vi "Autonomous Independent.vi"() -> ()   [LabVIEW 2016]
doc: "This VI is called when autonomous begins, and will automatically be terminated when autonomous ends. You can carry out timed or sensor driven robot movement independently without needing to return to the caller."
uses:
  <vilib>/Rock Robotics/Network Tables/NT Read Number.vi
  Global 2.vi
  Systems/Global 1.vi
panel:
  out "Numeric":i32=78
  out "Gyro":dbl=-0.15423582405
  in  "Oscillate effort":dbl=0.25 format="%#_13g"
  out "Auto Mode":dbl=2.0
  in  "Auton_Modes":T1(array[cluster])=[{"Actions"=[{"Effort"=0.55, "Duration"=3.5, "Action"=enum."Vision Correction", "Encoder"=0.0, "Condition"=FALSE}, {"Effort"=0.0, "Duration"=0.0, "Action"=enum."Nothing", "Encoder"=0.0, "Condition"=FALSE}]}, {"Actions"=[{"Effort"=0.53, "Duration"=1.0, "Action"=enum."Shoot", "Encoder"=6.462, "Condition"=TRUE}, {"Effort"=0.0, "Duration"=3.0, "Action"=enum."Index", "Encoder"=0.0, "Condition"=FALSE}, {"Effort"=0.3, "Duration"=2.0, "Action"=enum."Turn", "Encoder"=38.0, "Condition"=FALSE}, {"Effort"=0.3, "Duration"=5.0, "Action"=enum."Drive", "Encoder"=0.0, "Condition"=TRUE}, {"Effort"=0.25, "Duration"=0.0, "Action"=enum."Nothing", "Encoder"=57.0, "Condition"=FALSE}, {"Effort"=-0.25, "Duration"=0.0, "Action"=enum."Nothing", "Encoder"=0.0, "Condition"=FALSE}, {"Effort"=1.0, "Duration"=0.0, "Action"=enum."Nothing", "Encoder"=0.0, "Condition"=FALSE}, {"Effort"=0.25, "Duration"=0.0, "Action"=enum."Nothing", "Encoder"=0.0, "Condition"=FALSE}]}, {"Actions"=[{"Effort"=0.0, "Duration"=0.1, "Action"=enum."Drive Encoder Reset", "Encoder"=0.0, "Condition"=FALSE}, {"Effort"=0.0, "Duration"=0.1, "Action"=enum."Gyro Reset", "Encoder"=0.0, "Condition"=FALSE}, {"Effort"=0.3, "Duration"=2.5, "Action"=enum."Drive", "Encoder"=1000.0, "Condition"=TRUE}, {"Effort"=1.0, "Duration"=1.0, "Action"=enum."Gear0", "Encoder"=0.0, "Condition"=FALSE}, {"Effort"=1.0, "Duration"=0.0, "Action"=enum."Nothing", "Encoder"=0.0, "Condition"=FALSE}, {"Effort"=1.0, "Duration"=0.5, "Action"=enum."Nothing", "Encoder"=0.0, "Condition"=FALSE}, {"Effort"=0.0, "Duration"=0.0, "Action"=enum."Drive Encoder Reset", "Encoder"=0.0, "Condition"=FALSE}, {"Effort"=0.3, "Duration"=0.5, "Action"=enum."Nothing", "Encoder"=24.0, "Condition"=TRUE}, {"Effort"=0.0, "Duration"=0.0, "Action"=enum."Nothing", "Encoder"=0.0, "Condition"=FALSE}, {"Effort"=-0.2, "Duration"=2.0, "Action"=enum."Drive", "Encoder"=1000.0, "Condition"=TRUE}, {"Effort"=0.0, "Duration"=0.0, "Action"=enum."Drive Encoder Reset", "Encoder"=0.0, "Condition"=FALSE}, {"Effort"=-0.25, "Duration"=0.0, "Action"=enum."Nothing", "Encoder"=12.0, "Condition"=FALSE}]}, {"Actions"=[{"Effort"=0.0, "Duration"=0.1, "Action"=enum."Drive Encoder Reset", "Encoder"=6.462, "Condition"=FALSE}, {"Effort"=0.0, "Duration"=0.1, "Action"=enum."Gyro Reset", "Encoder"=0.0, "Condition"=FALSE}, {"Effort"=-0.25, "Duration"=1.0, "Action"=enum."Drive", "Encoder"=6.462, "Condition"=FALSE}, {"Effort"=0.0, "Duration"=0.1, "Action"=enum."Gyro Reset", "Encoder"=0.0, "Condition"=FALSE}, {"Effort"=-0.25, "Duration"=0.0, "Action"=enum."Turn", "Encoder"=0.0, "Condition"=FALSE}, {"Effort"=-0.25, "Duration"=0.0, "Action"=enum."Drive", "Encoder"=7.5, "Condition"=FALSE}, {"Effort"=-1.0, "Duration"=0.0, "Action"=enum."Gear0", "Encoder"=0.0, "Condition"=FALSE}, {"Effort"=0.25, "Duration"=0.0, "Action"=enum."Drive", "Encoder"=3.0, "Condition"=FALSE}]}, {"Actions"=[{"Effort"=0.0, "Duration"=0.1, "Action"=enum."Drive Encoder Reset", "Encoder"=6.462, "Condition"=FALSE}, {"Effort"=0.0, "Duration"=0.1, "Action"=enum."Gyro Reset", "Encoder"=0.0, "Condition"=FALSE}, {"Effort"=-0.25, "Duration"=1.0, "Action"=enum."Drive", "Encoder"=6.462, "Condition"=FALSE}, {"Effort"=0.0, "Duration"=0.1, "Action"=enum."Gyro Reset", "Encoder"=0.0, "Condition"=FALSE}, {"Effort"=-0.25, "Duration"=0.0, "Action"=enum."Turn", "Encoder"=0.0, "Condition"=FALSE}, {"Effort"=-0.25, "Duration"=0.0, "Action"=enum."Drive", "Encoder"=7.5, "Condition"=FALSE}, {"Effort"=-1.0, "Duration"=0.0, "Action"=enum."Gear0", "Encoder"=0.0, "Condition"=FALSE}, {"Effort"=0.25, "Duration"=0.0, "Action"=enum."Drive", "Encoder"=3.0, "Condition"=FALSE}]}, {"Actions"=[{"Effort"=0.0, "Duration"=0.1, "Action"=enum."Drive Encoder Reset", "Encoder"=0.0, "Condition"=FALSE}, {"Effort"=0.0, "Duration"=0.1, "Action"=enum."Gyro Reset", "Encoder"=0.0, "Condition"=FALSE}, {"Effort"=0.25, "Duration"=1.0, "Action"=enum."Drive", "Encoder"=6.462, "Condition"=FALSE}, {"Effort"=1.0, "Duration"=0.1, "Action"=enum."Gyro Reset", "Encoder"=0.0, "Condition"=FALSE}, {"Effort"=0.25, "Duration"=0.0, "Action"=enum."Turn", "Encoder"=0.0, "Condition"=FALSE}, {"Effort"=0.25, "Duration"=0.0, "Action"=enum."Drive", "Encoder"=7.5, "Condition"=FALSE}, {"Effort"=1.0, "Duration"=0.0, "Action"=enum."Gear0", "Encoder"=0.0, "Condition"=FALSE}, {"Effort"=-0.25, "Duration"=0.0, "Action"=enum."Drive", "Encoder"=3.0, "Condition"=FALSE}]}, {"Actions"=[{"Effort"=0.0, "Duration"=0.1, "Action"=enum."Nothing", "Encoder"=0.0, "Condition"=FALSE}, {"Effort"=0.0, "Duration"=0.1, "Action"=enum."Gyro Reset", "Encoder"=0.0, "Condition"=FALSE}, {"Effort"=0.25, "Duration"=5.0, "Action"=enum."Drive", "Encoder"=60000.0, "Condition"=TRUE}, {"Effort"=0.75, "Duration"=1.0, "Action"=enum."Nothing", "Encoder"=0.0, "Condition"=FALSE}, {"Effort"=0.0, "Duration"=1.0, "Action"=enum."Nothing", "Encoder"=0.0, "Condition"=FALSE}, {"Effort"=0.0, "Duration"=0.0, "Action"=enum."Nothing", "Encoder"=0.0, "Condition"=FALSE}]}, {"Actions"=[{"Effort"=0.0, "Duration"=0.5, "Action"=enum."Drive Encoder Reset", "Encoder"=0.0, "Condition"=FALSE}, {"Effort"=0.55, "Duration"=4.25, "Action"=enum."Gyro Reset", "Encoder"=0.0, "Condition"=FALSE}, {"Effort"=-0.5, "Duration"=0.0, "Action"=enum."Drive", "Encoder"=46.0, "Condition"=FALSE}, {"Effort"=0.3, "Duration"=1.0, "Action"=enum."Nothing", "Encoder"=0.0, "Condition"=FALSE}, {"Effort"=0.3, "Duration"=2.0, "Action"=enum."Vision Correction", "Encoder"=76.6, "Condition"=FALSE}, {"Effort"=-0.25, "Duration"=1.0, "Action"=enum."Drive", "Encoder"=18.5, "Condition"=TRUE}, {"Effort"=1.0, "Duration"=0.0, "Action"=enum."Gear0", "Encoder"=0.0, "Condition"=FALSE}, {"Effort"=0.3, "Duration"=1.3, "Action"=enum."Drive", "Encoder"=30.0, "Condition"=TRUE}, {"Effort"=0.0, "Duration"=0.0, "Action"=enum."Nothing", "Encoder"=0.0, "Condition"=FALSE}, {"Effort"=0.03, "Duration"=0.0, "Action"=enum."Turn", "Encoder"=0.0, "Condition"=FALSE}, {"Effort"=0.0, "Duration"=0.0, "Action"=enum."Drive", "Encoder"=0.0, "Condition"=FALSE}]}, {"Actions"=[{"Effort"=0.0, "Duration"=0.0, "Action"=enum."Nothing", "Encoder"=0.0, "Condition"=FALSE}]}, {"Actions"=[{"Effort"=0.0, "Duration"=2.5, "Action"=enum."Shoot", "Encoder"=0.0, "Condition"=FALSE}, {"Effort"=0.0, "Duration"=5.0, "Action"=enum."Index", "Encoder"=0.0, "Condition"=FALSE}, {"Effort"=0.25, "Duration"=3.5, "Action"=enum."Nothing", "Encoder"=88.0, "Condition"=FALSE}, {"Effort"=1.0, "Duration"=1.0, "Action"=enum."Nothing", "Encoder"=0.0, "Condition"=FALSE}, {"Effort"=1.0, "Duration"=1.0, "Action"=enum."Nothing", "Encoder"=0.0, "Condition"=FALSE}, {"Effort"=1.0, "Duration"=0.5, "Action"=enum."Nothing", "Encoder"=0.0, "Condition"=FALSE}, {"Effort"=0.0, "Duration"=0.0, "Action"=enum."Nothing", "Encoder"=0.0, "Condition"=FALSE}, {"Effort"=-0.25, "Duration"=0.0, "Action"=enum."Nothing", "Encoder"=3.0, "Condition"=FALSE}, {"Effort"=0.0, "Duration"=0.0, "Action"=enum."Nothing", "Encoder"=0.0, "Condition"=FALSE}, {"Effort"=0.25, "Duration"=0.0, "Action"=enum."Nothing", "Encoder"=24.0, "Condition"=FALSE}, {"Effort"=0.0, "Duration"=0.0, "Action"=enum."Nothing", "Encoder"=0.0, "Condition"=FALSE}, {"Effort"=-0.25, "Duration"=0.0, "Action"=enum."Nothing", "Encoder"=12.0, "Condition"=FALSE}]}, {"Actions"=[{"Effort"=0.0, "Duration"=0.1, "Action"=enum."Drive Encoder Reset", "Encoder"=0.0, "Condition"=FALSE}, {"Effort"=0.0, "Duration"=1.0, "Action"=enum."Gyro Reset", "Encoder"=0.0, "Condition"=FALSE}, {"Effort"=0.3, "Duration"=1.4, "Action"=enum."Drive", "Encoder"=88.0, "Condition"=TRUE}, {"Effort"=0.3, "Duration"=4.0, "Action"=enum."Turn", "Encoder"=2.0, "Condition"=FALSE}, {"Effort"=1.0, "Duration"=1.0, "Action"=enum."Nothing", "Encoder"=0.0, "Condition"=FALSE}, {"Effort"=1.0, "Duration"=0.5, "Action"=enum."Nothing", "Encoder"=0.0, "Condition"=FALSE}, {"Effort"=0.0, "Duration"=0.0, "Action"=enum."Nothing", "Encoder"=0.0, "Condition"=FALSE}, {"Effort"=-0.25, "Duration"=0.0, "Action"=enum."Nothing", "Encoder"=3.0, "Condition"=FALSE}, {"Effort"=0.0, "Duration"=0.0, "Action"=enum."Nothing", "Encoder"=0.0, "Condition"=FALSE}, {"Effort"=0.25, "Duration"=0.0, "Action"=enum."Nothing", "Encoder"=24.0, "Condition"=FALSE}, {"Effort"=0.0, "Duration"=0.0, "Action"=enum."Nothing", "Encoder"=0.0, "Condition"=FALSE}, {"Effort"=-0.25, "Duration"=0.0, "Action"=enum."Nothing", "Encoder"=12.0, "Condition"=FALSE}]}, {"Actions"=[{"Effort"=0.0, "Duration"=1.0, "Action"=enum."Drive Encoder Reset", "Encoder"=0.0, "Condition"=FALSE}, {"Effort"=0.0, "Duration"=1.0, "Action"=enum."Shoot", "Encoder"=0.0, "Condition"=FALSE}, {"Effort"=0.25, "Duration"=5.0, "Action"=enum."Index", "Encoder"=88.0, "Condition"=FALSE}, {"Effort"=1.0, "Duration"=1.0, "Action"=enum."Nothing", "Encoder"=0.0, "Condition"=FALSE}, {"Effort"=1.0, "Duration"=1.0, "Action"=enum."Nothing", "Encoder"=0.0, "Condition"=FALSE}, {"Effort"=1.0, "Duration"=0.5, "Action"=enum."Nothing", "Encoder"=0.0, "Condition"=FALSE}, {"Effort"=0.0, "Duration"=0.0, "Action"=enum."Nothing", "Encoder"=0.0, "Condition"=FALSE}, {"Effort"=-0.25, "Duration"=0.0, "Action"=enum."Nothing", "Encoder"=3.0, "Condition"=FALSE}, {"Effort"=0.0, "Duration"=0.0, "Action"=enum."Nothing", "Encoder"=0.0, "Condition"=FALSE}, {"Effort"=0.25, "Duration"=0.0, "Action"=enum."Nothing", "Encoder"=24.0, "Condition"=FALSE}, {"Effort"=0.0, "Duration"=0.0, "Action"=enum."Nothing", "Encoder"=0.0, "Condition"=FALSE}, {"Effort"=-0.25, "Duration"=0.0, "Action"=enum."Nothing", "Encoder"=12.0, "Condition"=FALSE}]}, {"Actions"=[{"Effort"=0.0, "Duration"=0.1, "Action"=enum."Drive Encoder Reset", "Encoder"=0.0, "Condition"=FALSE}, {"Effort"=0.0, "Duration"=1.0, "Action"=enum."Gyro Reset", "Encoder"=0.0, "Condition"=FALSE}, {"Effort"=0.3, "Duration"=1.4, "Action"=enum."Drive", "Encoder"=88.0, "Condition"=TRUE}, {"Effort"=0.3, "Duration"=4.0, "Action"=enum."Turn", "Encoder"=0.0, "Condition"=FALSE}, {"Effort"=1.0, "Duration"=1.0, "Action"=enum."Nothing", "Encoder"=0.0, "Condition"=FALSE}, {"Effort"=1.0, "Duration"=0.5, "Action"=enum."Nothing", "Encoder"=0.0, "Condition"=FALSE}, {"Effort"=0.0, "Duration"=0.0, "Action"=enum."Nothing", "Encoder"=0.0, "Condition"=FALSE}, {"Effort"=0.3, "Duration"=0.5, "Action"=enum."Nothing", "Encoder"=24.0, "Condition"=TRUE}, {"Effort"=0.0, "Duration"=0.0, "Action"=enum."Nothing", "Encoder"=0.0, "Condition"=FALSE}, {"Effort"=-0.2, "Duration"=2.0, "Action"=enum."Nothing", "Encoder"=24.0, "Condition"=TRUE}, {"Effort"=0.0, "Duration"=0.0, "Action"=enum."Nothing", "Encoder"=0.0, "Condition"=FALSE}, {"Effort"=-0.25, "Duration"=0.0, "Action"=enum."Nothing", "Encoder"=12.0, "Condition"=FALSE}]}]
  # "Nothing"
  # "Boiler Right Right side gear"
  # "Middle Gear"
  # "Boiler Right Left Side Gear"
  # "Boiler Left RightSide Gear"
  # "Boiler Left Left Side Gear"
  # "Drive"
  # "Vision Correction"
  # "Hopper"
  # "10 ball"
  # "Farside"
  # "Boilerside-10 ball"
  # "Auto 5"
  # "Auto 6"
  # "Auto 6"
  # "Auto 7"
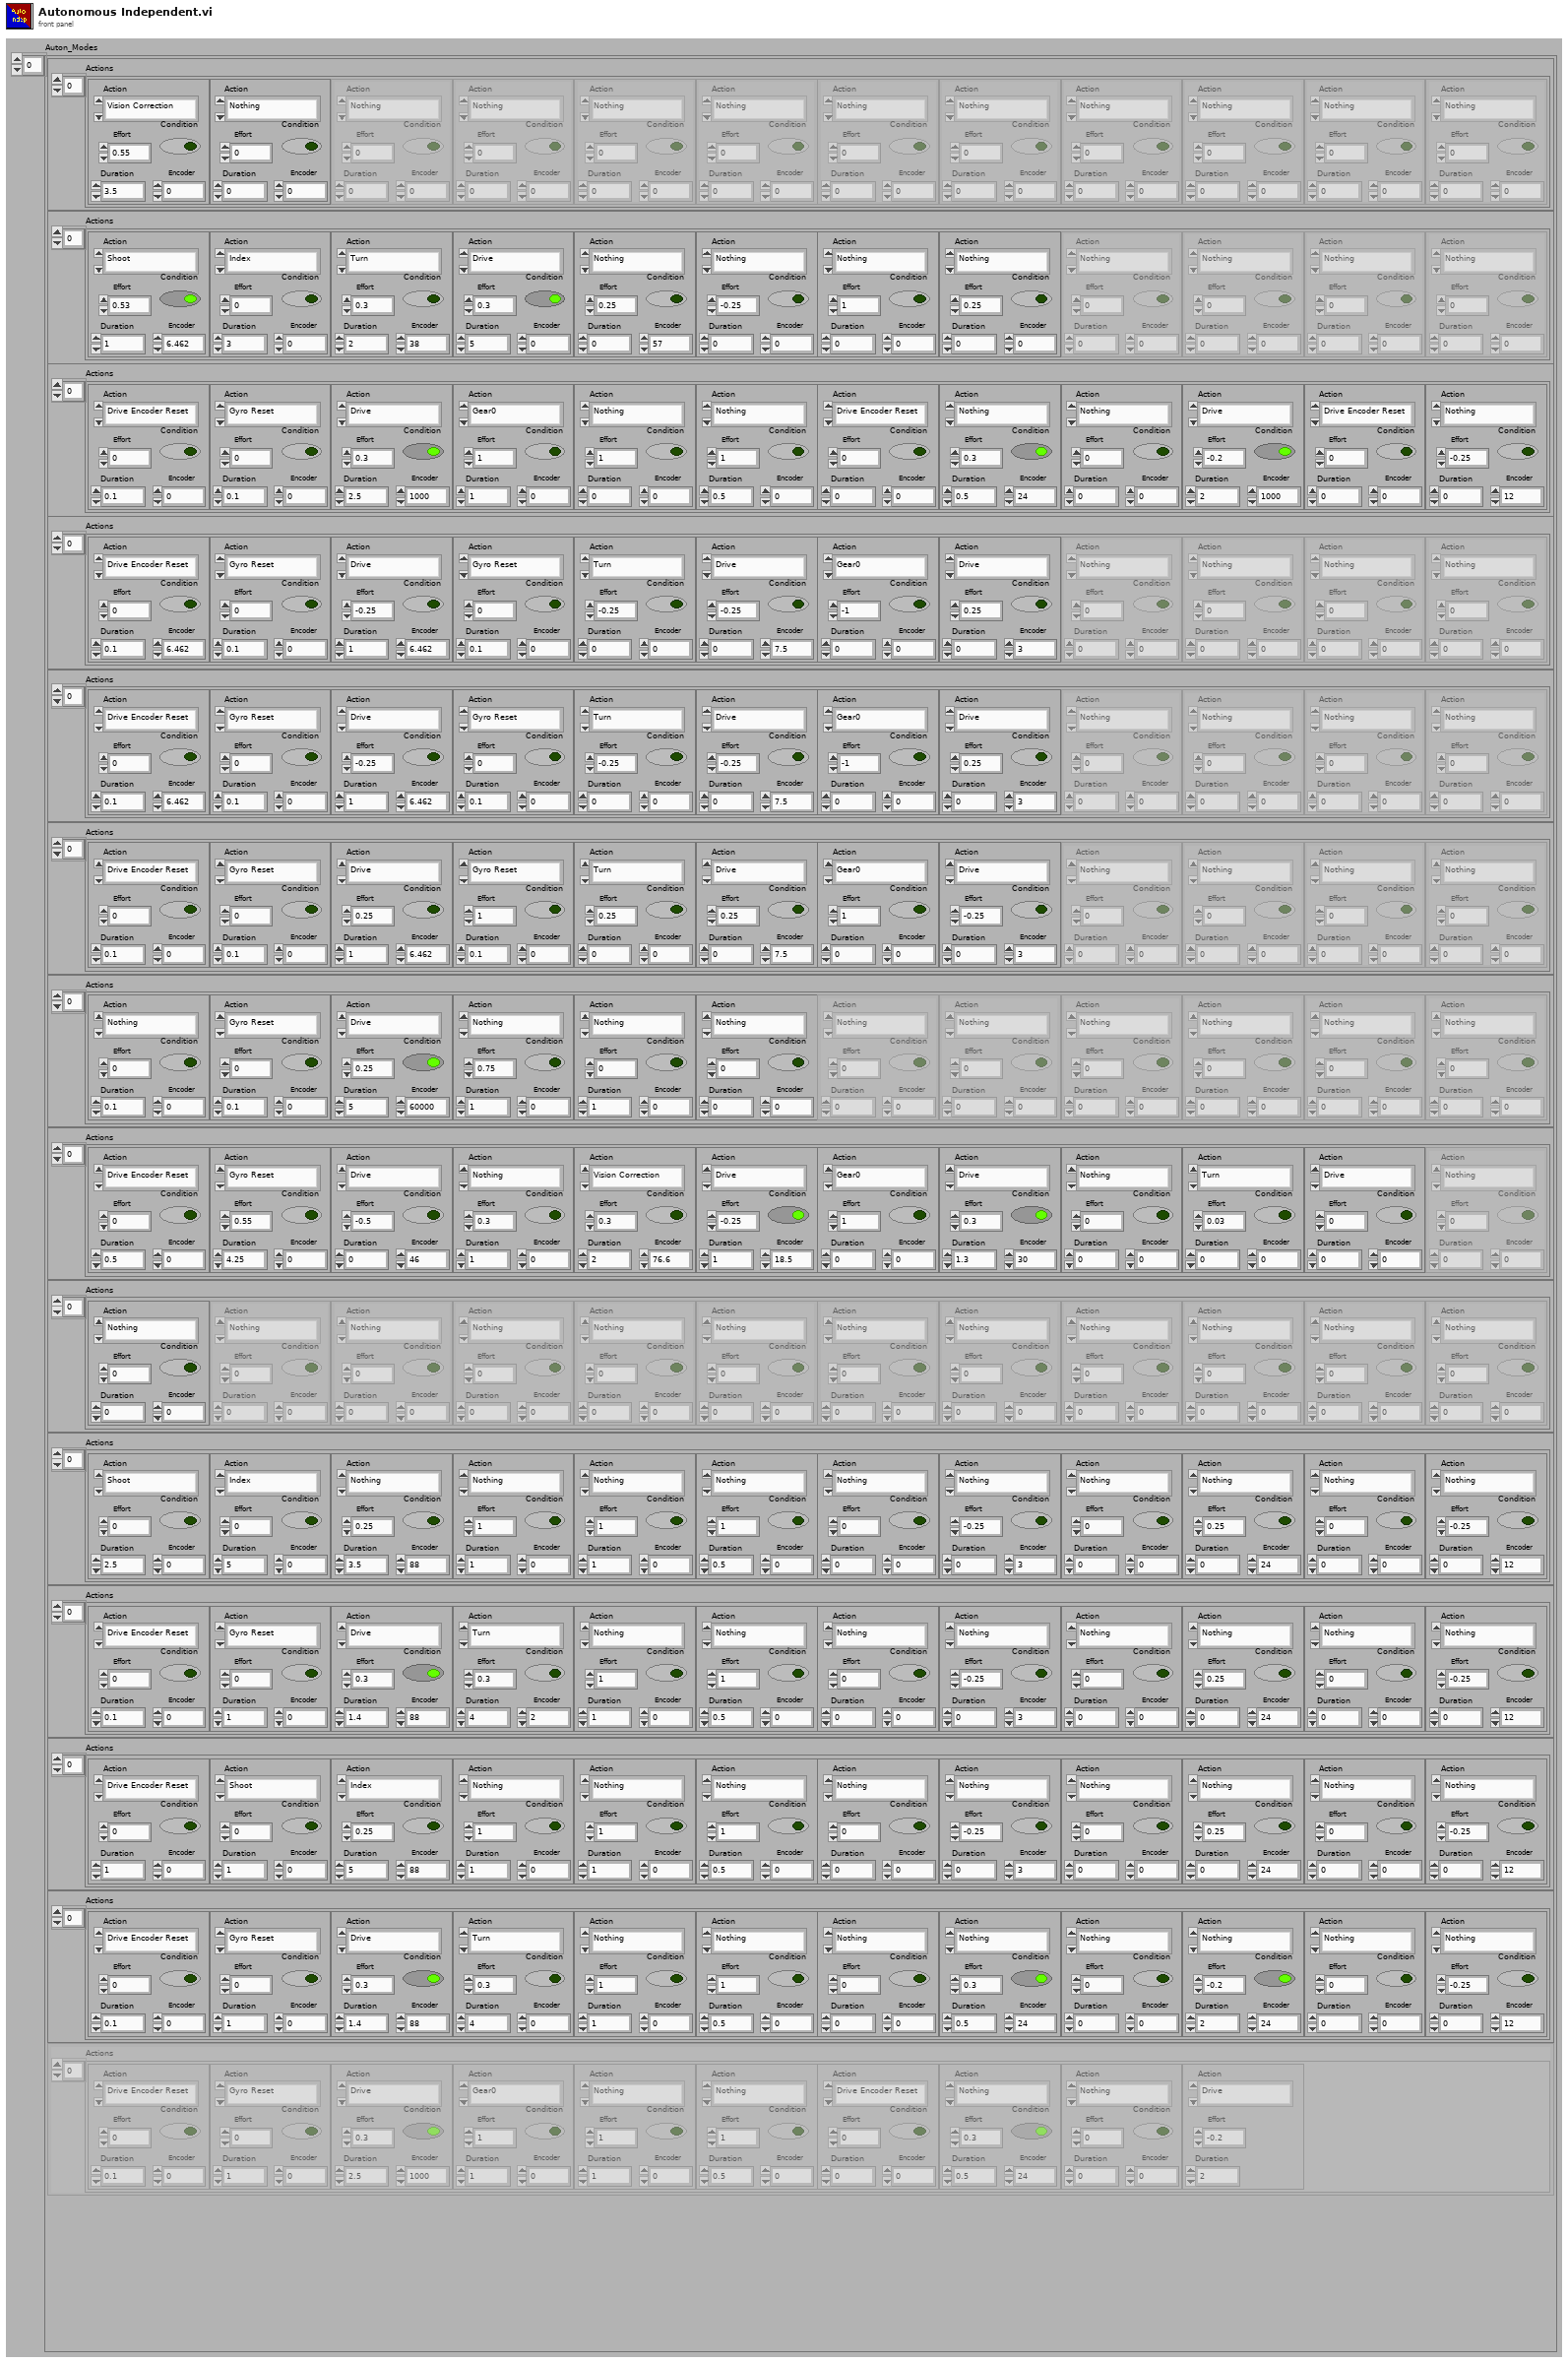
[diagram p1: front panel]
types:
  T1 = cluster{"Actions":cluster{"Effort":dbl, "Duration":dbl, "Action":enum16{"Nothing", "Drive", "Vision Correction", "Turn", "Gear0", "Gear1", "Climb", "Intake", "Index", "Shoot", "Test", "Drive Encoder Reset", "Gyro Reset"}, "Encoder":dbl, "Condition":bool}[]}[]
  T2 = cluster{"Actions":cluster{"Effort":dbl, "Duration":dbl, "Action":enum16{"Nothing", "Drive", "Vision Correction", "Turn", "Gear0", "Gear1", "Climb", "Intake", "Index", "Shoot", "Test", "Drive Encoder Reset", "Gyro Reset"}, "Encoder":dbl, "Condition":bool}[]}
  T3 = cluster{"Effort":dbl, "Duration":dbl, "Action":enum16{"Nothing", "Drive", "Vision Correction", "Turn", "Gear0", "Gear1", "Climb", "Intake", "Index", "Shoot", "Test", "Drive Encoder Reset", "Gyro Reset"}, "Encoder":dbl, "Condition":bool}[]
  T4 = enum16{"Nothing", "Drive", "Vision Correction", "Turn", "Gear0", "Gear1", "Climb", "Intake", "Index", "Shoot", "Test", "Drive Encoder Reset", "Gyro Reset"}
  T5 = typedef "WPI_MotorControlDeviceRef.ctl" = cluster{"DeviceStatus":errorcluster, "Type":T6, "PWM":cluster{"PWM Channel":T7, "DeadBand":T8}, "CAN":cluster{"Device Number":u8, "SetOutput VI Ref":variant, "GetOutput VI Ref":variant, "Enable VI Ref":variant, "Disable VI Ref":variant, "Data":variant}, "Invert":bool}
  T6 = typedef "WPI_MotorControlType.ctl" = enum16{"PWM", "CAN"}
  T7 = typedef "FPGA_DIOPWMChannel.ctl" = enum8{"PWM 0", "PWM 1", "PWM 2", "PWM 3", "PWM 4", "PWM 5", "PWM 6", "PWM 7", "PWM 8", "PWM 9", "PWM MXP 0", "PWM MXP 1", "PWM MXP 2", "PWM MXP 3", "PWM MXP 4", "PWM MXP 5", "PWM MXP 6", "PWM MXP 7", "PWM MXP 8", "PWM MXP 9", "Invalid"}
  T8 = typedef "WPI_PWMDeadband.ctl" = cluster{"Name":string, "maxPositivePwm":i32, "minPositivePwm":i32, "centerPwm":i32, "maxNegativePwm":i32, "minNegativePwm":i32, "angularRange":u16}
  T9 = typedef "WPI_CANTalonSRX_GlobalStatus.ctl" = cluster{"Applied Throttle":dbl, "Module Enabled":bool, "CAN Error":errorcluster, "Closed Loop Error":dbl, "Forward Limit Switch Closed":bool, "Reverse Limit Switch Closed":bool, "Sensor Position":dbl, "Sensor Velocity":dbl, "Current":dbl, "Sticky Fault - Over Temp":bool, "Sticky Fault - Under Voltage":bool, "Sticky Fault - Forward Limit":bool, "Sticky Fault - Reverse Limit":bool, "Sticky Fault - Forward Soft Limit":bool, "Sticky Fault - Reverse Soft Limit":bool, "Brake is Enabled":bool, "Encoder Position":dbl, "Encoder Velocity":dbl, "Encoder Index Count":dbl, "Encoder A Pin State":bool, "Encoder B Pin State":bool, "Encoder Index Pin State":bool, "Analog In":dbl, "Analog In Velocity":dbl, "Temperature (C)":dbl, "Battery Voltage":dbl, "Control 5 Is Supported":bool, "Current Profile Slot Select":dbl, "Pos Div 8":bool, "Vel Div 4":bool, "Pulse Width Position":i32, "Pulse Width Velocity":i32, "Pulse Width Rise To Rise (us)":i32, "Pulse Width Rise To Fall (us)":i32, "Mot Prof Active Is Under Run":bool, "Mot Prof Active Has Under Run":bool, "Mot Prof Active Is Last":bool, "Mot Prof Active Velocity Only":bool, "Mot Prof Active Is Valid":bool, "Mot Prof Buffer Is Full":bool, "Mot Prof Active Profile Slot Select":i32, "Mot Prof NextID":i32, "Mot Prof Count":i32, "Mot Prof Active Velocity":dbl, "Mot Prof Active Position":dbl, "Mot Prof Output Enable":i32}
  T10 = typedef "WPI_GyroDevRef.ctl" = cluster{"DevStatus":errorcluster, "Analog Channel":T11, "Offset":dbl, "Gain (VoltsPerDegree/Second)":dbl, "Gyro Type":enum16{"Analog", "XRS450"}, "Handle":i32, "SPI Bus":T12, "Device Found":bool, "Sample Rate":dbl, "Calibrate On Open":bool}
  T11 = typedef "FPGA_AIChannel.ctl" = enum8{"AI 0", "AI 1", "AI 2", "AI 3", "AI MXP 0", "AI MXP 1", "AI MXP 2", "AI MXP 3", "Invalid"}
  T12 = typedef "spi_bus.ctl" = enum16{"SPI On-Board, CS0", "SPI On-Board, CS1", "SPI On-Board, CS2", "SPI On-Board, CS3", "SPI MXP", "Invalid"}
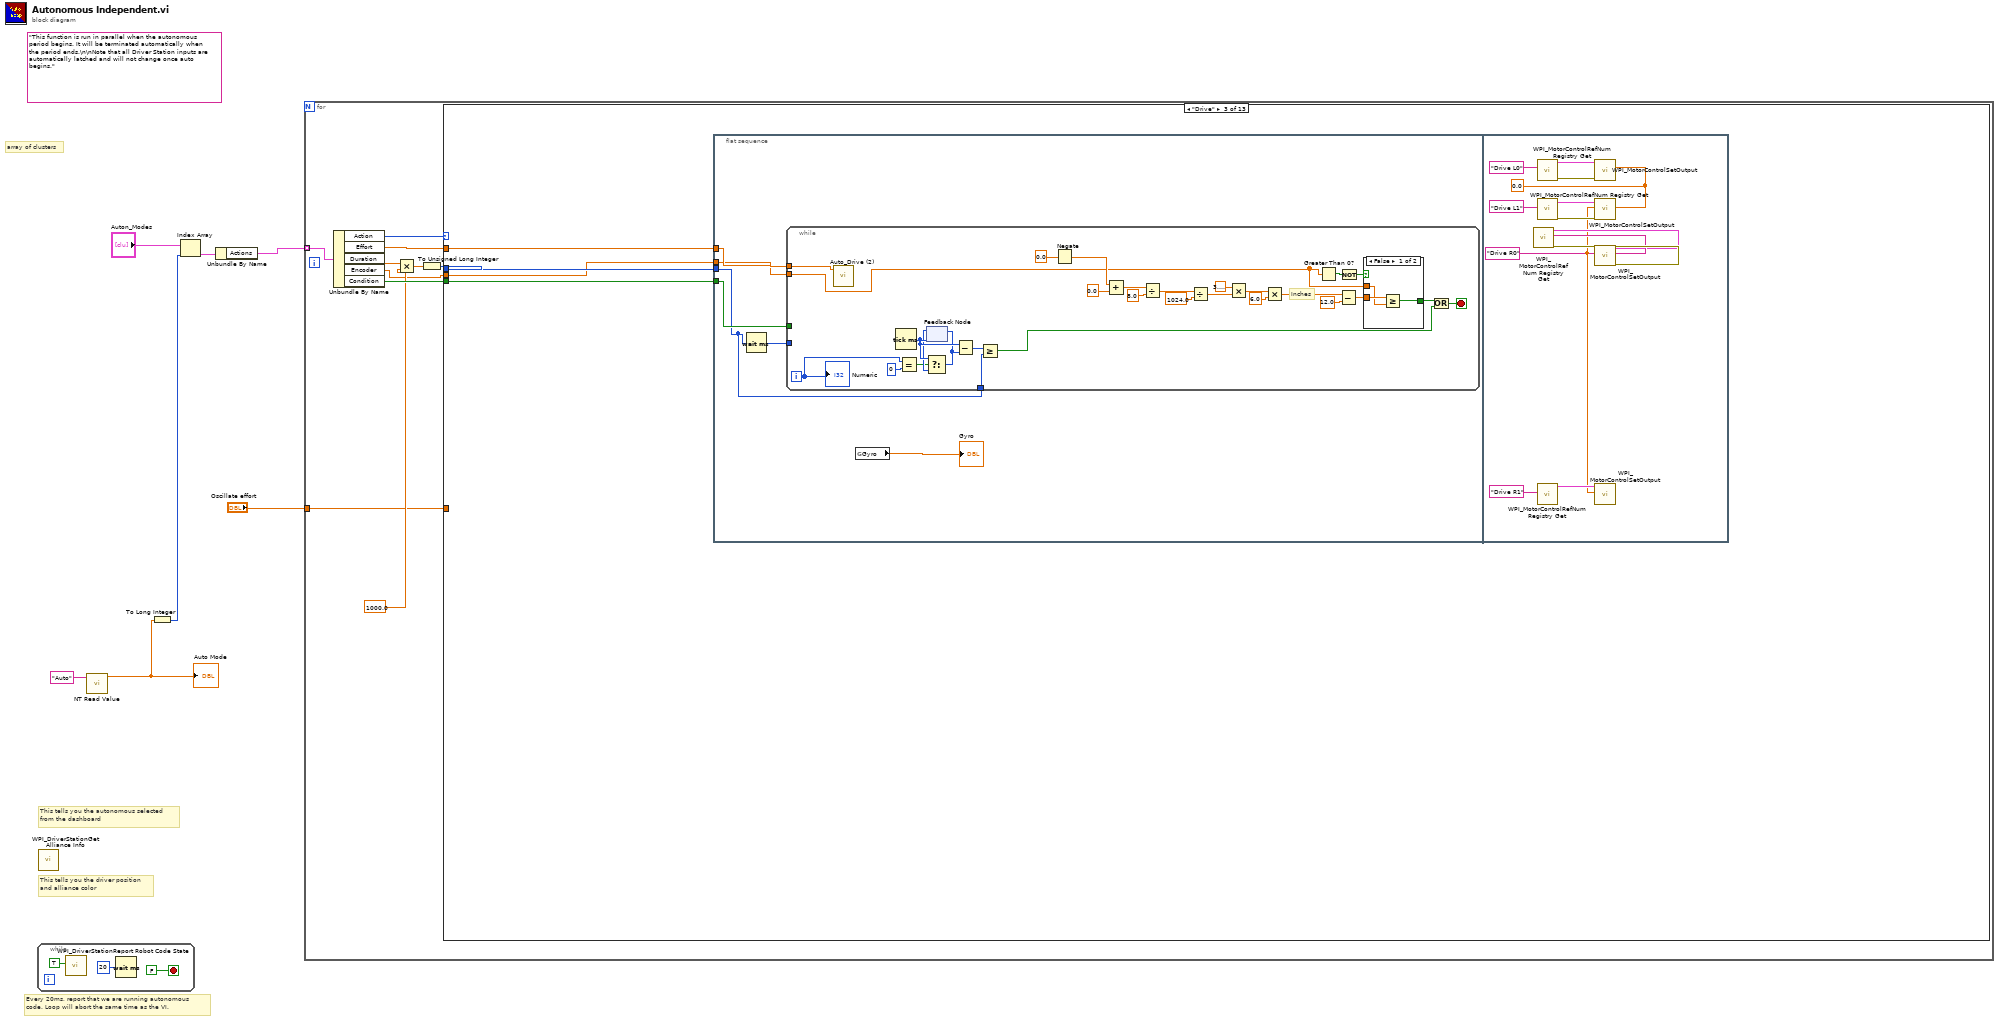
[diagram p0: block diagram]
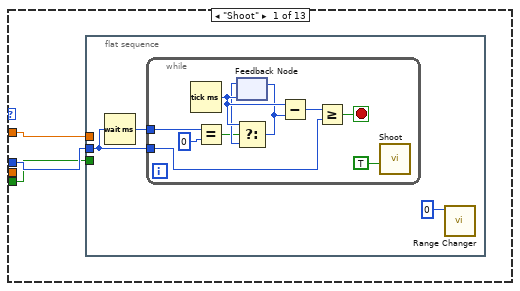
[diagram p2: hidden frame]
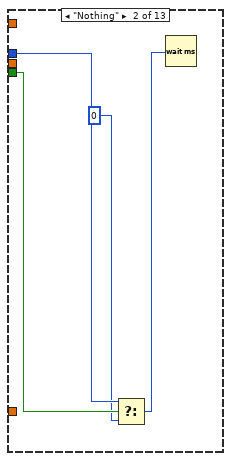
[diagram p3: hidden frame]
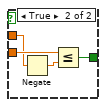
[diagram p4: hidden frame]
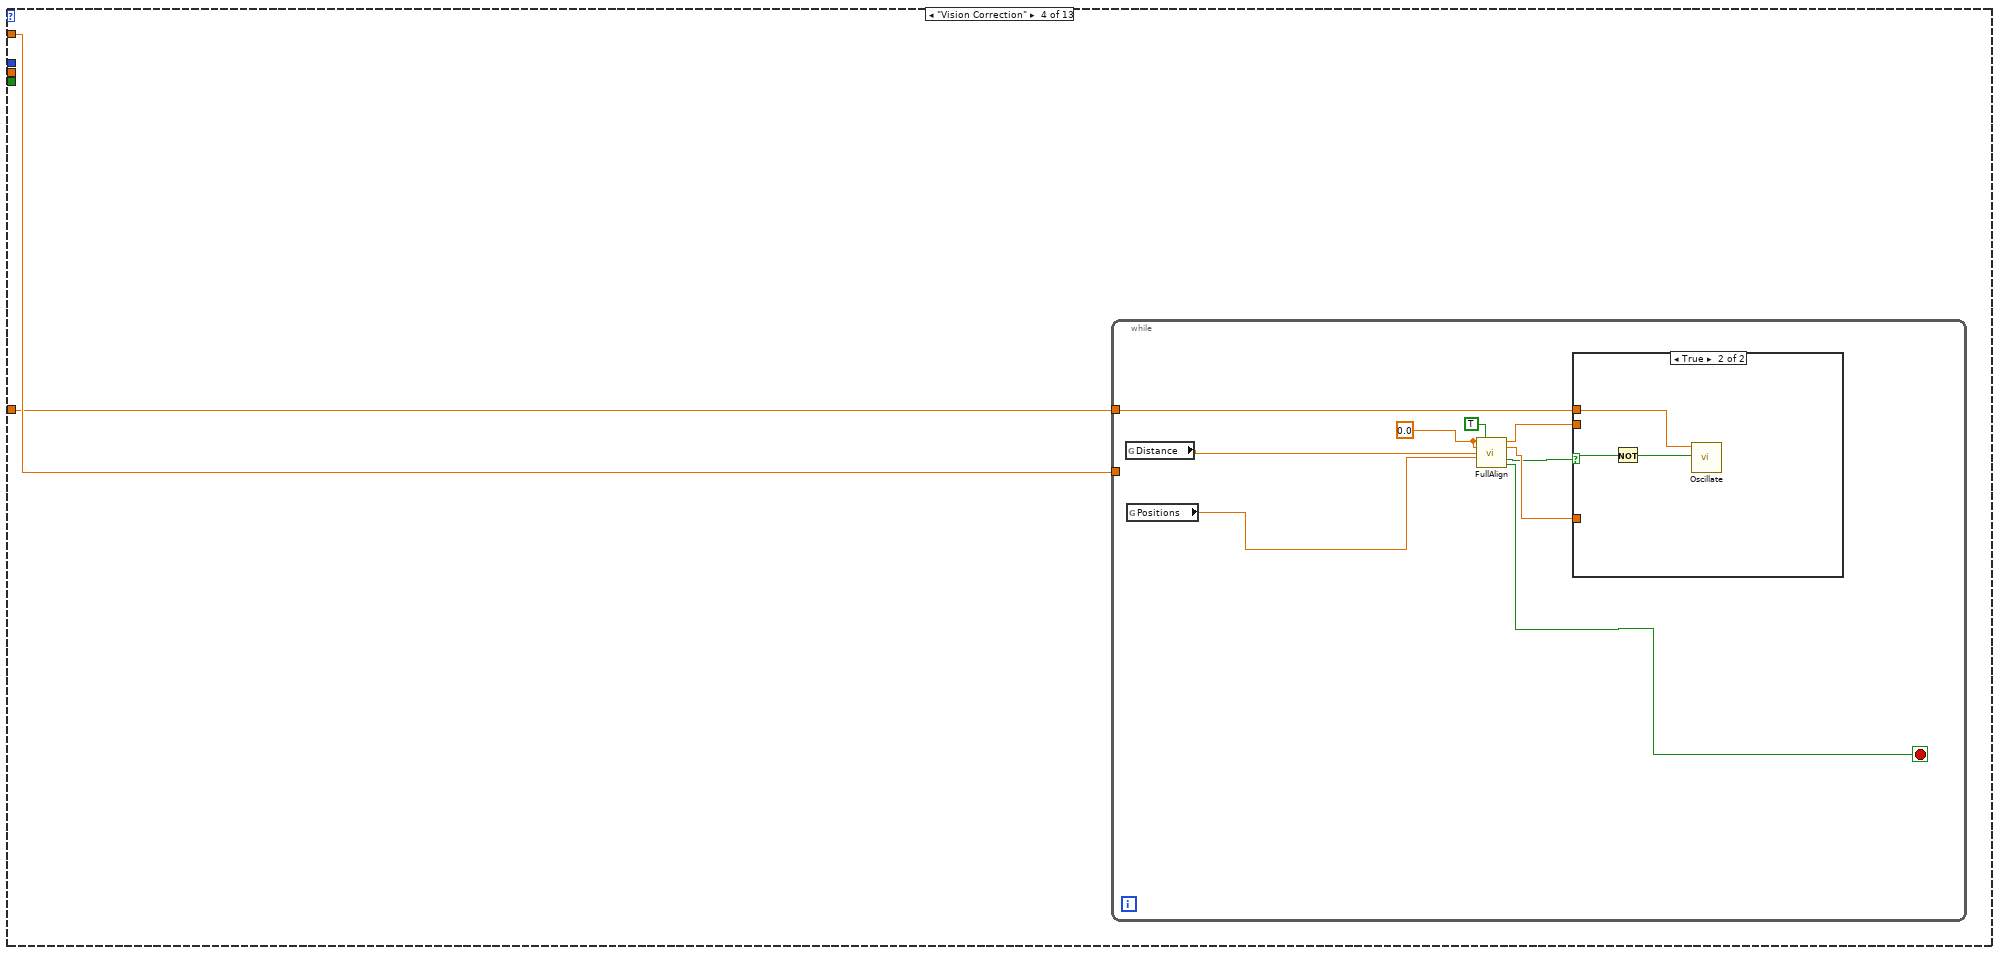
[diagram p5: hidden frame]
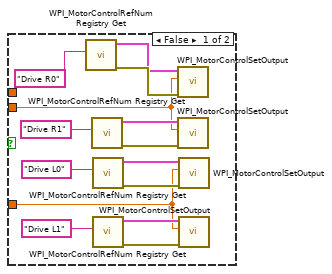
[diagram p6: hidden frame]
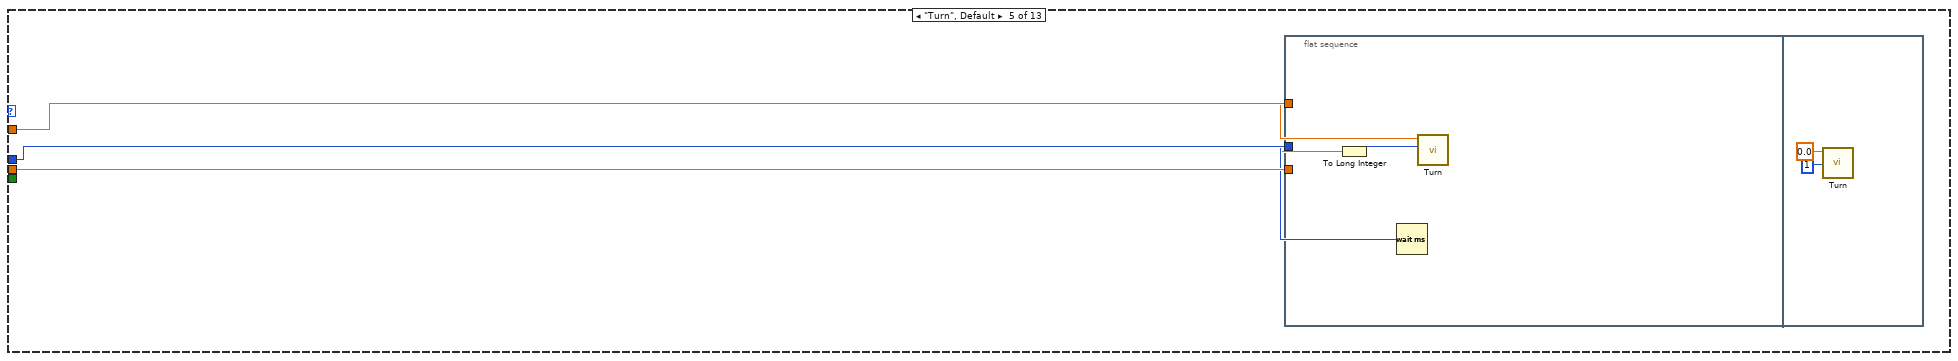
[diagram p7: hidden frame]
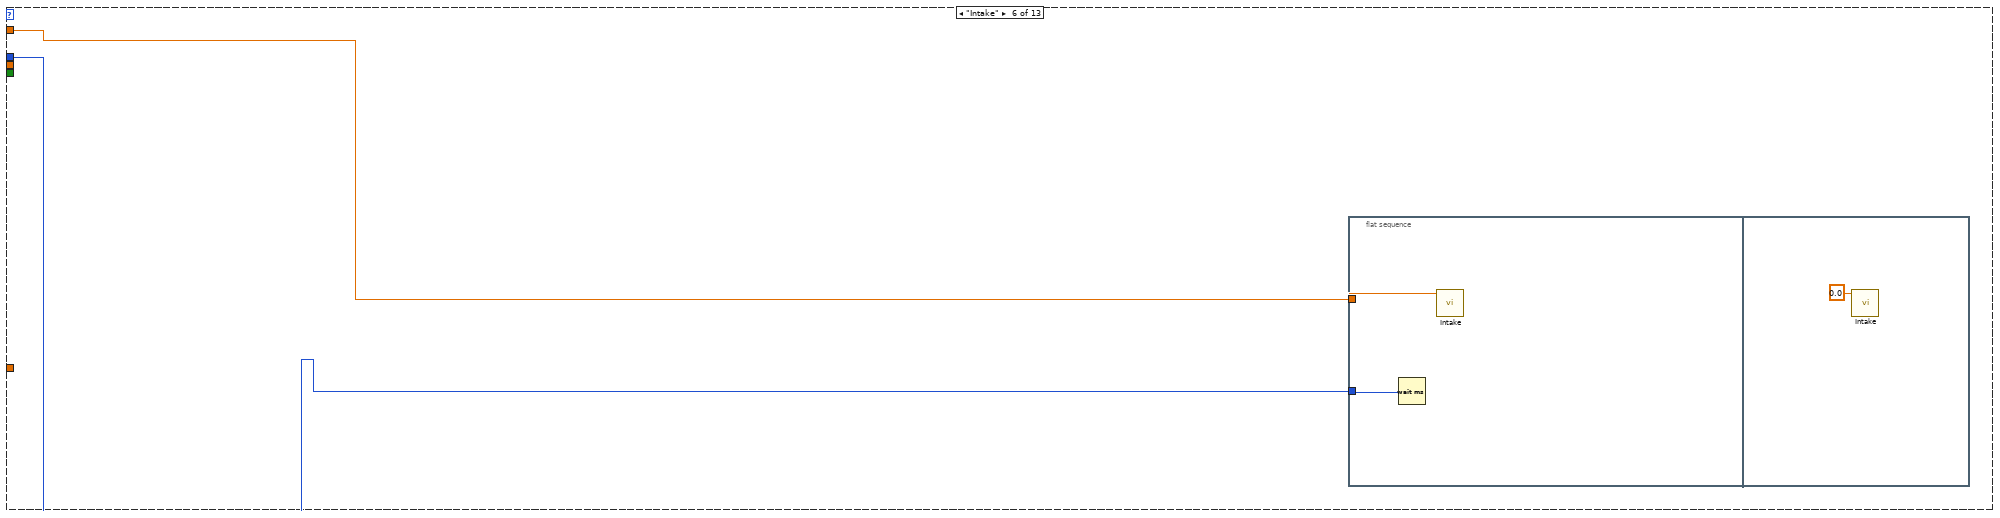
[diagram p8: hidden frame]
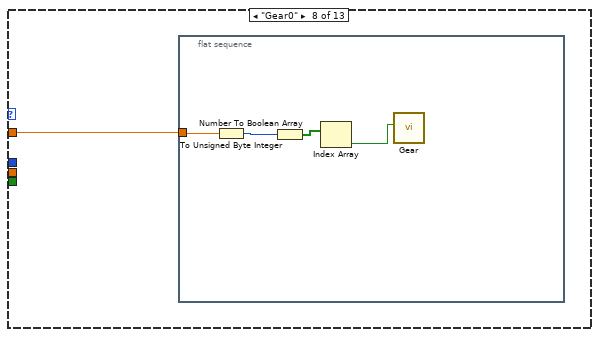
[diagram p10: hidden frame]
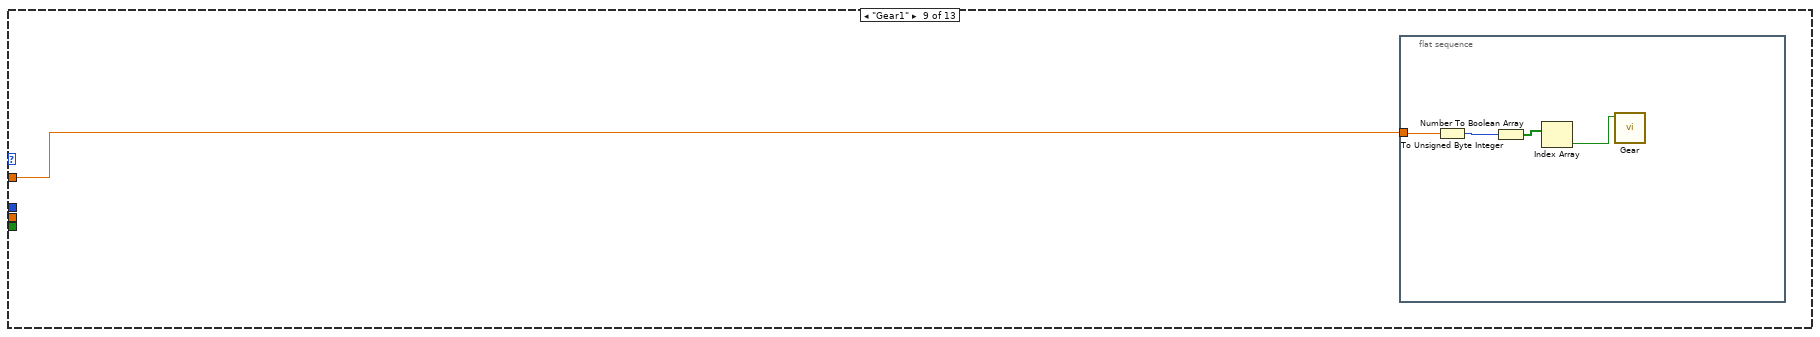
[diagram p11: hidden frame]
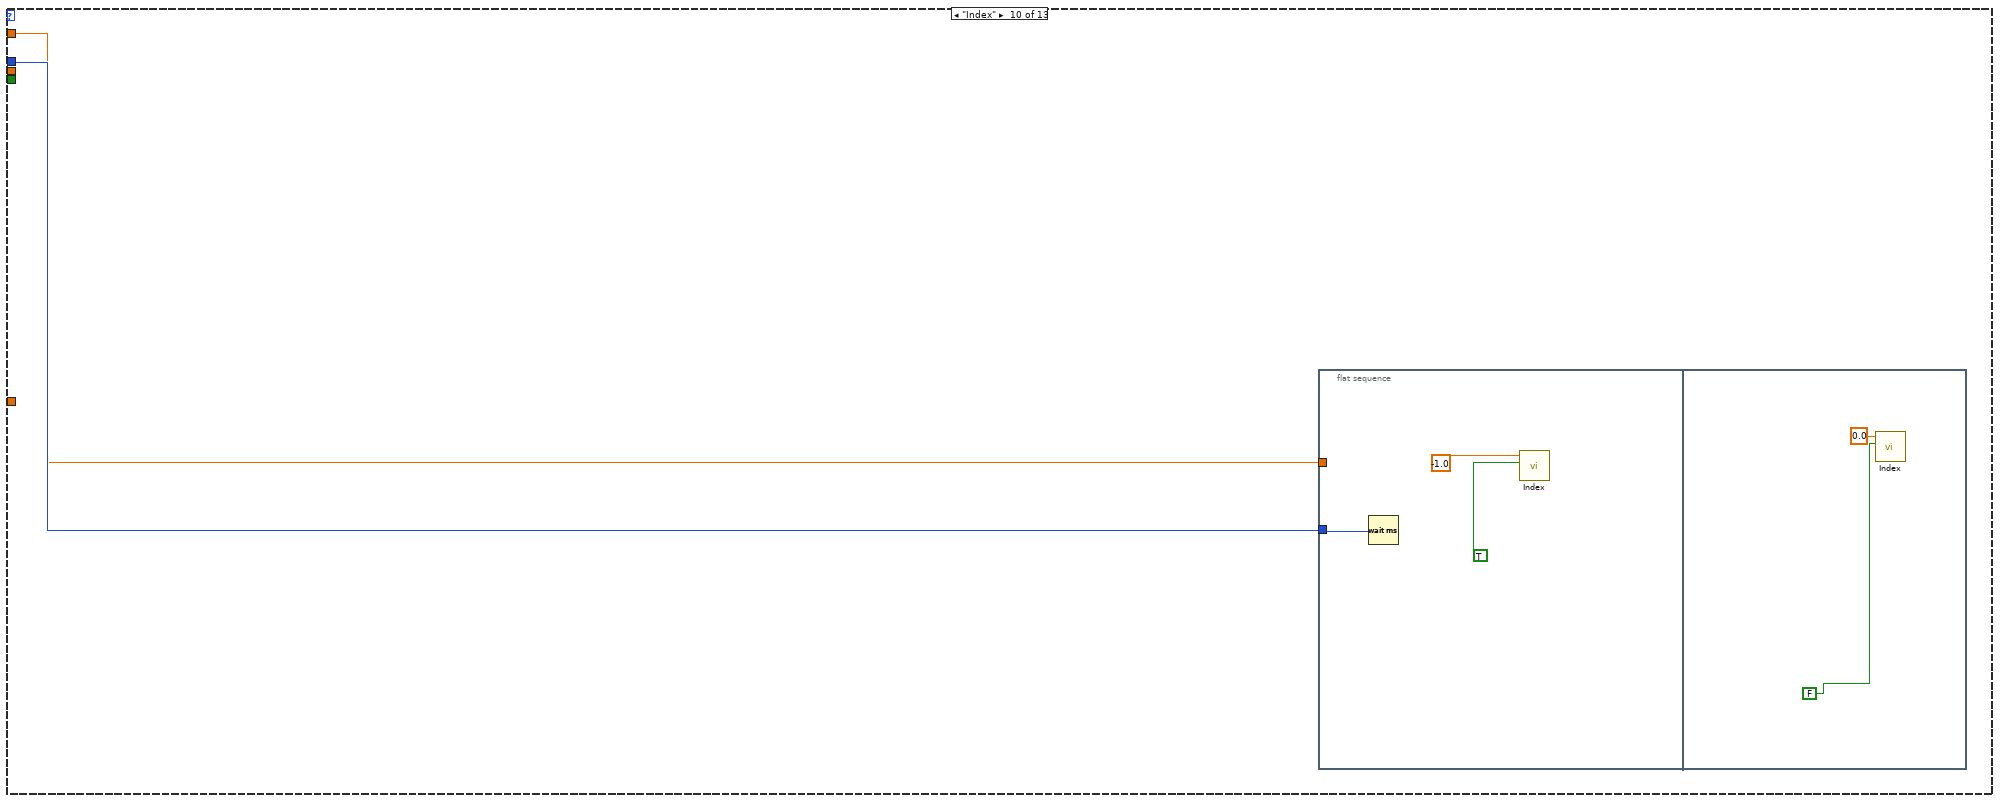
[diagram p12: hidden frame]
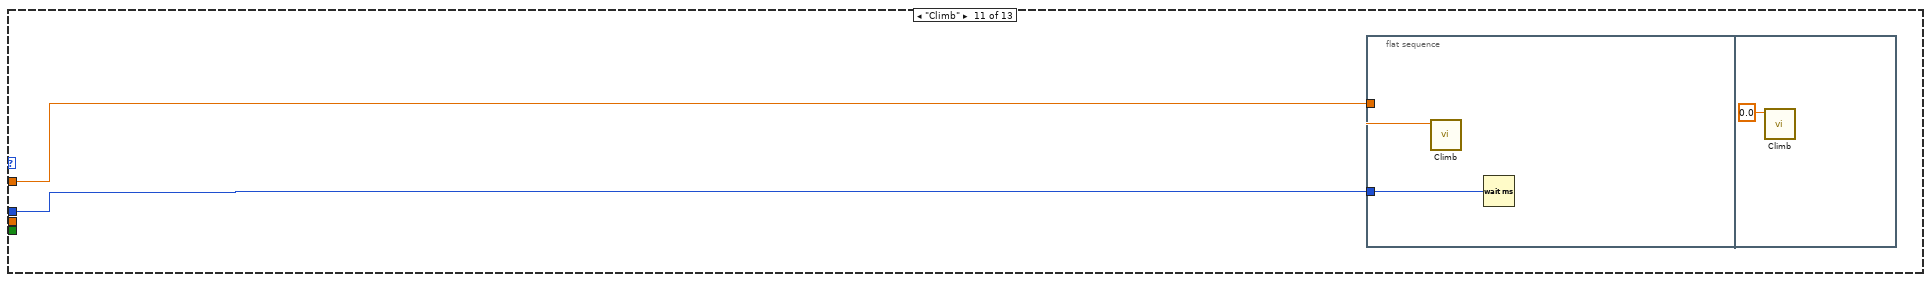
[diagram p13: hidden frame]
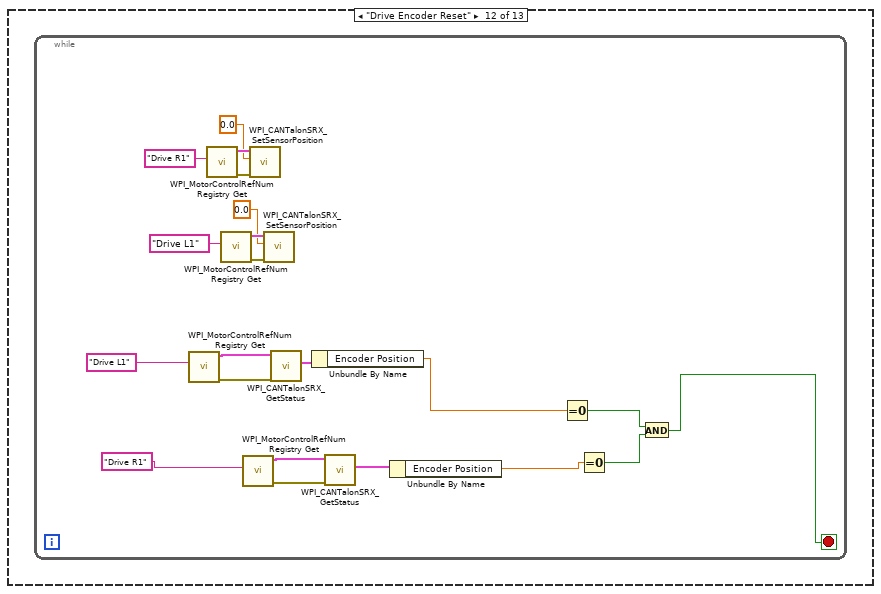
[diagram p14: hidden frame]
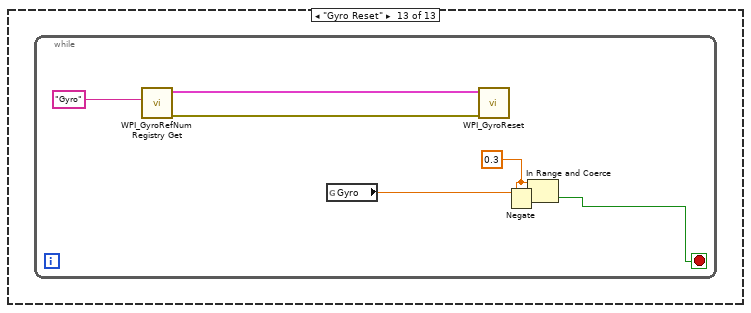
[diagram p15: hidden frame]
diagram:
  (unwired) "This function is run in parallel when the autonomous period begins. It will be terminated automatically when the period ends.\n\nNote that all Driver Station inputs are automatically latched and will not change once auto begins."
  # "This tells you the autonomous selected\nfrom the dashboard"
  # "array of clusters"
  # "Every 20ms, report that we are running autonomous\ncode. Loop will abort the same time as the VI."
  # "This tells you the driver position\nand alliance color"
  n1 = while {
    stop <- FALSE stop-if-true
    n2 = call <vilib>:"WPI_DriverStationReport Robot Code State.vi"("Autonomous"=TRUE) -> ()  [unwired: 10 in, 1 out]
    n3 = Wait (ms)(milliseconds to wait=u32 20) -> ()  [unwired: 1 out]
  }
  n4 = call <vilib>:"WPI_DriverStationGet Alliance Info.vi"() -> ()  [unwired: 12 out]
  n5 = call-poly <vilib>:"NT Read Value.vi"("Name"="Auto") -> ("Numeric"=w2:dbl)  [unwired: 9 in, 1 out]
  "Auto Mode" <- w2
  n6 = To Long Integer(number=w2) -> (32bit integer=w4:i32)
  n7 = Index Array(array="Auton_Modes", index=w4) -> (element=w6:T2)
  n8 = Unbundle By Name(w6) -> ("Actions"=w7:T3)
  n9 = for {
    tunnel: w7 -> [w20] mode=indexing
    tunnel: "Oscillate effort" -> [w11]
    n10 = Unbundle By Name(w20) -> ("Action"=w19:T4, "Effort"=w18:dbl, "Duration"=w17:dbl, "Encoder"=w12:dbl, "Condition"=w14:bool)
    n11 = Multiply(x=w17, y=1000.0) -> (x*y=w16:dbl)
    n12 = To Unsigned Long Integer(number=w16) -> (unsigned 32bit integer=w15:u32)
    n13 = case shown="\"Drive\"" w19 {
      tunnel: w18 -> [w23 _ w44 w100 w129 w137 _ w141 w146 w151 w159 _ _]
      tunnel: w15 -> [w22 w39 w43 _ w128 w136 _ _ _ w152 w158 _ _]
      tunnel: w14 -> [w21 w40 w42 _ _ _ _ _ _ _ _ _ _]
      tunnel: w12 -> [_ _ w41 _ w127 _ _ _ _ _ _ _ _]
      tunnel: w11 -> [_ _ _ w99 _ _ _ _ _ _ _ _ _]
      frame "Shoot" {
        n14 = flat-sequence {
          tunnel: w23 -> [_]
          tunnel: w22 -> [w24]
          tunnel: w21 -> [_]
          frame #0 {
            n15 = Wait (ms)(milliseconds to wait=w24) -> (millisecond timer value=w25:u32)
            n16 = while {
              tunnel: w25 -> [w28]
              tunnel: w24 -> [w27]
              stop <- w29 stop-if-true
              n17 = Tick Count (ms)() -> (millisecond timer value=w35:u32)
              n18 = Equal?(x=w28, y=0) -> (x = y?=w33:bool)
              n19 = feedback #1(w35) -> (w34:u32)
              n20 = Select(t=w35, s=w33, f=w34) -> (s? t:f=w31:u32)
              n21 = feedback-in #1(w31) -> ()
              n22 = Subtract(x=w35, y=w31) -> (x-y=w30:u32)
              n23 = Greater Or Equal?(x=w30, y=w27) -> (x >= y?=w29:bool)
              n24 = call "Shoot.vi"("Shoot"=TRUE) -> ()  [unwired: 10 in]
            }
            n25 = call "Range Changer.vi"("POV"=i16 0) -> ()  [unwired: 10 in, 1 out]
          }
        }
      }
      frame "Nothing" {
        n26 = Select(t=w39, s=w40, f=u32 0) -> (s? t:f=w37:u32)
        n27 = Wait (ms)(milliseconds to wait=w37) -> ()  [unwired: 1 out]
      }
      frame "Drive" {
        n28 = flat-sequence {
          tunnel: w44 -> [w50]
          tunnel: w43 -> [w45]
          tunnel: w42 -> [w48]
          tunnel: w41 -> [w49]
          frame #0 {
            n29 = Wait (ms)(milliseconds to wait=w45) -> (millisecond timer value=w46:u32)
            n30 = while {
              tunnel: w50 -> [w79]
              tunnel: w49 -> [w62]
              tunnel: w48 -> [_]
              tunnel: w46 -> [_]
              tunnel: w45 -> [w53]
              i -> [w51]
              stop <- w63 stop-if-true
              # "Inches"
              n31 = call "Auto_Drive (2).vi"("Drive Effort"=w79) -> ()  [unwired: 11 in]
              n32 = Tick Count (ms)() -> (millisecond timer value=w59:u32)
              n33 = Equal?(x=w51, y=0) -> (x = y?=w57:bool)
              n34 = feedback #2(w59) -> (w58:u32)
              n35 = Select(t=w59, s=w57, f=w58) -> (s? t:f=w55:u32)
              n36 = feedback-in #2(w55) -> ()
              n37 = Subtract(x=w59, y=w55) -> (x-y=w54:u32)
              n38 = Greater Or Equal?(x=w54, y=w53) -> (x >= y?=w52:bool)
              n39 = Negate(x=0.0) -> (-x=w78:dbl)
              n40 = Add(x=w78, y=0.0) -> (x+y=w77:dbl)
              n41 = Divide(x=w77, y=8.0) -> (x/y=w75:dbl)
              n42 = Divide(x=w75, y=1024.0) -> (x/y=w73:dbl)
              n43 = Multiply(x=3.141592653589793, y=w73) -> (x*y=w71:dbl)
              n44 = Multiply(x=w71, y=6.0) -> (x*y=w69:dbl)
              n45 = Greater Than 0?(x=w62) -> (x > 0?=w66:bool)
              n46 = Subtract(x=w69, y=12.0) -> (x-y=w67:dbl)
              n47 = Not(x=w66) -> (.not. x?=w64:bool)
              n48 = case shown="False" w64 {
                tunnel: [w81 w86] -> w65
                tunnel: w67 -> [w82 w84]
                tunnel: w62 -> [w80 w83]
                frame False {
                  n49 = Greater Or Equal?(x=w82, y=w80) -> (x >= y?=w81:bool)
                }
                frame True {
                  n50 = Negate(x=w83) -> (-x=w85:dbl)
                  n51 = Less Or Equal?(x=w84, y=w85) -> (x <= y?=w86:bool)
                }
              }
              n52 = Or(x=w65, y=w52) -> (x .or. y?=w63:bool)
              "Numeric" <- w51
            }
            n53 = global read "Global 2.vi" "Gyro"() -> (→"Gyro":dbl)
          }
          frame #1 {
            w87 = 0.0 ("Drive L")
            n54 = call <vilib>:"WPI_MotorControlRefNum Registry Get.vi"("refnum name"="Drive R0") -> ("error out"=w92:errorcluster, "MotorControlDevRef"=w88:T5)  [unwired: 9 in]
            n55 = call <vilib>:"WPI_MotorControlRefNum Registry Get.vi"("refnum name"="Drive L0") -> ("error out"=w93:errorcluster, "MotorControlDevRef"=w94:T5)  [unwired: 9 in]
            n56 = call <vilib>:"WPI_MotorControlRefNum Registry Get.vi"("refnum name"="Drive L1") -> ("error out"=w97:errorcluster, "MotorControlDevRef"=w96:T5)  [unwired: 9 in]
            n57 = call <vilib>:"WPI_MotorControlRefNum Registry Get.vi"("refnum name"="Drive R1") -> ("MotorControlDevRef"=w90:T5)  [unwired: 9 in, 1 out]
            n58 = call <vilib>:"WPI_MotorControlSetOutput.vi"("error in (no error)"=w93, "Output"=w87, "MotorControlDevRef"=w94) -> ()  [unwired: 6 in, 3 out]
            n59 = call <vilib>:"WPI_MotorControlSetOutput.vi"("error in (no error)"=w97, "Output"=w87, "MotorControlDevRef"=w96) -> ()  [unwired: 6 in, 3 out]
            n60 = call <vilib>:"WPI_MotorControlSetOutput.vi"("error in (no error)"=w92, "Output"=w87, "MotorControlDevRef"=w88) -> ()  [unwired: 6 in, 3 out]
            n61 = call <vilib>:"WPI_MotorControlSetOutput.vi"("Output"=w87, "MotorControlDevRef"=w90) -> ()  [unwired: 7 in, 3 out]
          }
        }
      }
      frame "Vision Correction" {
        n62 = while {
          tunnel: w100 -> [_]
          tunnel: w99 -> [w102]
          stop <- w104 stop-if-true
          w107 = 0.0
          n63 = global read "Global 1.vi" "Distance"() -> (w106:dbl)
          n64 = global read "Global 1.vi" "Positions"() -> (w105:dbl)
          n65 = call "FullAlign.vi"("Joystick 0"=w107, "Button"=TRUE, "Joystick 1"=w107, "Distance"=w106, "Angle"=w105) -> ("Right Motor"=w109:dbl, "Left Motor"=w108:dbl, "Not In Sight?"=w103:bool, "In Range?"=w104:bool)  [unwired: 7 in]
          n66 = case shown="True" w103 {
            selector: w103 -> [_ w126]
            tunnel: w109 -> [w111 _]
            tunnel: w108 -> [w110 _]
            tunnel: w102 -> [_ w124]
            frame False {
              n67 = call <vilib>:"WPI_MotorControlRefNum Registry Get.vi"("refnum name"="Drive R0") -> ("error out"=w117:errorcluster, "MotorControlDevRef"=w113:T5)  [unwired: 9 in]
              n68 = call <vilib>:"WPI_MotorControlRefNum Registry Get.vi"("refnum name"="Drive R1") -> ("error out"=w112:errorcluster, "MotorControlDevRef"=w115:T5)  [unwired: 9 in]
              n69 = call <vilib>:"WPI_MotorControlRefNum Registry Get.vi"("refnum name"="Drive L0") -> ("error out"=w118:errorcluster, "MotorControlDevRef"=w119:T5)  [unwired: 9 in]
              n70 = call <vilib>:"WPI_MotorControlRefNum Registry Get.vi"("refnum name"="Drive L1") -> ("error out"=w122:errorcluster, "MotorControlDevRef"=w121:T5)  [unwired: 9 in]
              n71 = call <vilib>:"WPI_MotorControlSetOutput.vi"("error in (no error)"=w117, "Output"=w111, "MotorControlDevRef"=w113) -> ()  [unwired: 6 in, 3 out]
              n72 = call <vilib>:"WPI_MotorControlSetOutput.vi"("error in (no error)"=w112, "Output"=w111, "MotorControlDevRef"=w115) -> ()  [unwired: 6 in, 3 out]
              n73 = call <vilib>:"WPI_MotorControlSetOutput.vi"("error in (no error)"=w118, "Output"=w110, "MotorControlDevRef"=w119) -> ()  [unwired: 6 in, 3 out]
              n74 = call <vilib>:"WPI_MotorControlSetOutput.vi"("error in (no error)"=w122, "Output"=w110, "MotorControlDevRef"=w121) -> ()  [unwired: 6 in, 3 out]
            }
            frame True {
              n75 = Not(x=w126) -> (.not. x?=w125:bool)
              n76 = call "Oscillate.vi"("Target In Sight?"=w125, "Effort"=w124) -> ()  [unwired: 10 in]
            }
          }
        }
      }
      frame "Turn", Default {
        n77 = flat-sequence {
          tunnel: w129 -> [w133]
          tunnel: w128 -> [w132]
          tunnel: w127 -> [w130]
          frame #0 {
            n78 = To Long Integer(number=w130) -> (32bit integer=w131:i32)
            n79 = Wait (ms)(milliseconds to wait=w132) -> ()  [unwired: 1 out]
            n80 = call "Turn.vi"("mode"=w131, "Effort"=w133) -> ()  [unwired: 10 in]
          }
          frame #1 {
            n81 = call "Turn.vi"("mode"=1, "Effort"=0.0) -> ()  [unwired: 10 in]
          }
        }
      }
      frame "Intake" {
        n82 = flat-sequence {
          tunnel: w137 -> [w139]
          tunnel: w136 -> [w138]
          frame #0 {
            n83 = Wait (ms)(milliseconds to wait=w138) -> ()  [unwired: 1 out]
            n84 = call "Intake.vi"("Effort"=w139) -> ()  [unwired: 11 in]
          }
          frame #1 {
            n85 = call "Intake.vi"("Effort"=0.0) -> ()  [unwired: 11 in]
          }
        }
      }
      frame "Test" {
      }
      frame "Gear0" {
        n86 = flat-sequence {
          tunnel: w141 -> [w145]
          frame #0 {
            n87 = To Unsigned Byte Integer(number=w145) -> (unsigned 8bit integer=w144:u8)
            n88 = Number To Boolean Array(number=w144) -> (Boolean array=w143:bool[])
            n89 = Index Array(array=w143) -> (element=w142:bool)  [unwired: 1 in]
            n90 = call "Gear.vi"("Gear0?"=w142) -> ()  [unwired: 11 in]
          }
        }
      }
      frame "Gear1" {
        n91 = flat-sequence {
          tunnel: w146 -> [w150]
          frame #0 {
            n92 = To Unsigned Byte Integer(number=w150) -> (unsigned 8bit integer=w149:u8)
            n93 = Number To Boolean Array(number=w149) -> (Boolean array=w148:bool[])
            n94 = Index Array(array=w148) -> (element=w147:bool)  [unwired: 1 in]
            n95 = call "Gear.vi"("Gear1?"=w147) -> ()  [unwired: 11 in]
          }
        }
      }
      frame "Index" {
        n96 = flat-sequence {
          tunnel: w152 -> [w153]
          tunnel: w151 -> [_]
          frame #0 {
            n97 = Wait (ms)(milliseconds to wait=w153) -> ()  [unwired: 1 out]
            n98 = call "Index.vi"("Shoot"=TRUE ("Override?"), "Output"=-1.0) -> ()  [unwired: 10 in]
          }
          frame #1 {
            n99 = call "Index.vi"("Shoot"=FALSE ("Override?"), "Output"=0.0) -> ()  [unwired: 10 in]
          }
        }
      }
      frame "Climb" {
        n100 = flat-sequence {
          tunnel: w159 -> [w161]
          tunnel: w158 -> [w160]
          frame #0 {
            n101 = call "Climb.vi"("Effort"=w161) -> ()  [unwired: 11 in]
            n102 = Wait (ms)(milliseconds to wait=w160) -> ()  [unwired: 1 out]
          }
          frame #1 {
            n103 = call "Climb.vi"("Effort"=0.0) -> ()  [unwired: 11 in]
          }
        }
      }
      frame "Drive Encoder Reset" {
        n104 = while {
          stop <- w163 stop-if-true
          n105 = call <vilib>:"WPI_MotorControlRefNum Registry Get.vi"("refnum name"="Drive L1") -> ("error out"=w173:errorcluster, "MotorControlDevRef"=w168:T5)  [unwired: 9 in]
          n106 = call <vilib>:"WPI_MotorControlRefNum Registry Get.vi"("refnum name"="Drive R1") -> ("error out"=w178:errorcluster, "MotorControlDevRef"=w177:T5)  [unwired: 9 in]
          n107 = call <vilib>:"WPI_MotorControlRefNum Registry Get.vi"("refnum name"="Drive L1") -> ("error out"=w180:errorcluster, "MotorControlDevRef"=w181:T5)  [unwired: 9 in]
          n108 = call <vilib>:"WPI_MotorControlRefNum Registry Get.vi"("refnum name"="Drive R1") -> ("error out"=w170:errorcluster, "MotorControlDevRef"=w169:T5)  [unwired: 9 in]
          n109 = call <vilib>:"WPI_CANTalonSRX_SetSensorPosition.vi"("error in (no error)"=w178, "New Sensor Position"=0.0, "CAN Talon SRX Ref"=w177) -> ()  [unwired: 7 in, 2 out]
          n110 = call <vilib>:"WPI_CANTalonSRX_SetSensorPosition.vi"("error in (no error)"=w180, "New Sensor Position"=0.0, "CAN Talon SRX Ref"=w181) -> ()  [unwired: 7 in, 2 out]
          n111 = call <vilib>:"WPI_CANTalonSRX_GetStatus.vi"("error in (no error)"=w173, "CAN Talon SRX Ref"=w168) -> ("Talon SRX Status"=w171:T9)  [unwired: 7 in, 2 out]
          n112 = Unbundle By Name(w171) -> ("Encoder Position"=w166:dbl)
          n113 = call <vilib>:"WPI_CANTalonSRX_GetStatus.vi"("error in (no error)"=w170, "CAN Talon SRX Ref"=w169) -> ("Talon SRX Status"=w172:T9)  [unwired: 7 in, 2 out]
          n114 = Unbundle By Name(w172) -> ("Encoder Position"=w167:dbl)
          n115 = Equal To 0?(x=w166) -> (x = 0?=w165:bool)
          n116 = Equal To 0?(x=w167) -> (x = 0?=w164:bool)
          n117 = And(x=w165, y=w164) -> (x .and. y?=w163:bool)
        }
      }
      frame "Gyro Reset" {
        n118 = while {
          stop <- w184 stop-if-true
          w187 = 0.3
          n119 = call <vilib>:"WPI_GyroRefNum Registry Get.vi"("refnum name"="Gyro") -> ("error out"=w189:errorcluster, "GyroDevRef"=w190:T10)  [unwired: 9 in]
          n120 = global read "Global 2.vi" "Gyro"() -> (w185:dbl)
          n121 = call <vilib>:"WPI_GyroReset.vi"("error in"=w189, "GyroDevRef"=w190) -> ()  [unwired: 8 in, 2 out]
          n122 = Negate(x=w187) -> (-x=w186:dbl)
          n123 = In Range and Coerce(upper limit=w187, x=w185, lower limit=w186) -> (In Range?=w184:bool)  [unwired: 1 out]
        }
      }
    }
  }
